vi "ServoControl_myrio_v3.vi"() -> ()   [LabVIEW 2019]
uses:
  <vilib>/Platform/TimedLoop/XDataNode/timing_clust.ctl
  <vilib>/Platform/TimedLoop/XDataNode/nitl_modes.ctl
  <vilib>/Platform/TimedLoop/XDataNode/wakeup.ctl
  <vilib>/Instr/_visa.llb/VISA Configure Serial Port (Instr).vi
  <vilib>/platform/TimedLoop/XDataNode/XDataNode.xnode
  <vilib>/Platform/TimedLoop/XDataNode/XDNodeRunTimeDep.lvlib
panel:
  in  "plot freq.":i32=100
  out "Position Graph":cluster{dbl[], dbl[]}[](graph)
  in  "stop":bool
  in  "const(f)/sine(t)":bool
  out "iteration":i32
  out "time":dbl
  out "sine position":dbl
  in  "Period":i64=5
  out "Position Chart":cluster{dbl, dbl}(graph)
  out "read from visa":string
  out "write to visa":string
  in  "VISA resource name":refnum<visa-resource-name>
  in  "baud rate (9600)":u32=500000
  in  "stop":bool
  out "read buffer 2":string
  in  "write buffer":string
  in  "Boolean 2":bool
  in  "const posotion":dbl
  out "error out":errorcluster
  # "white:write\nred:read"
  # "visa setting"
  # "measure time"
  # "status setting"
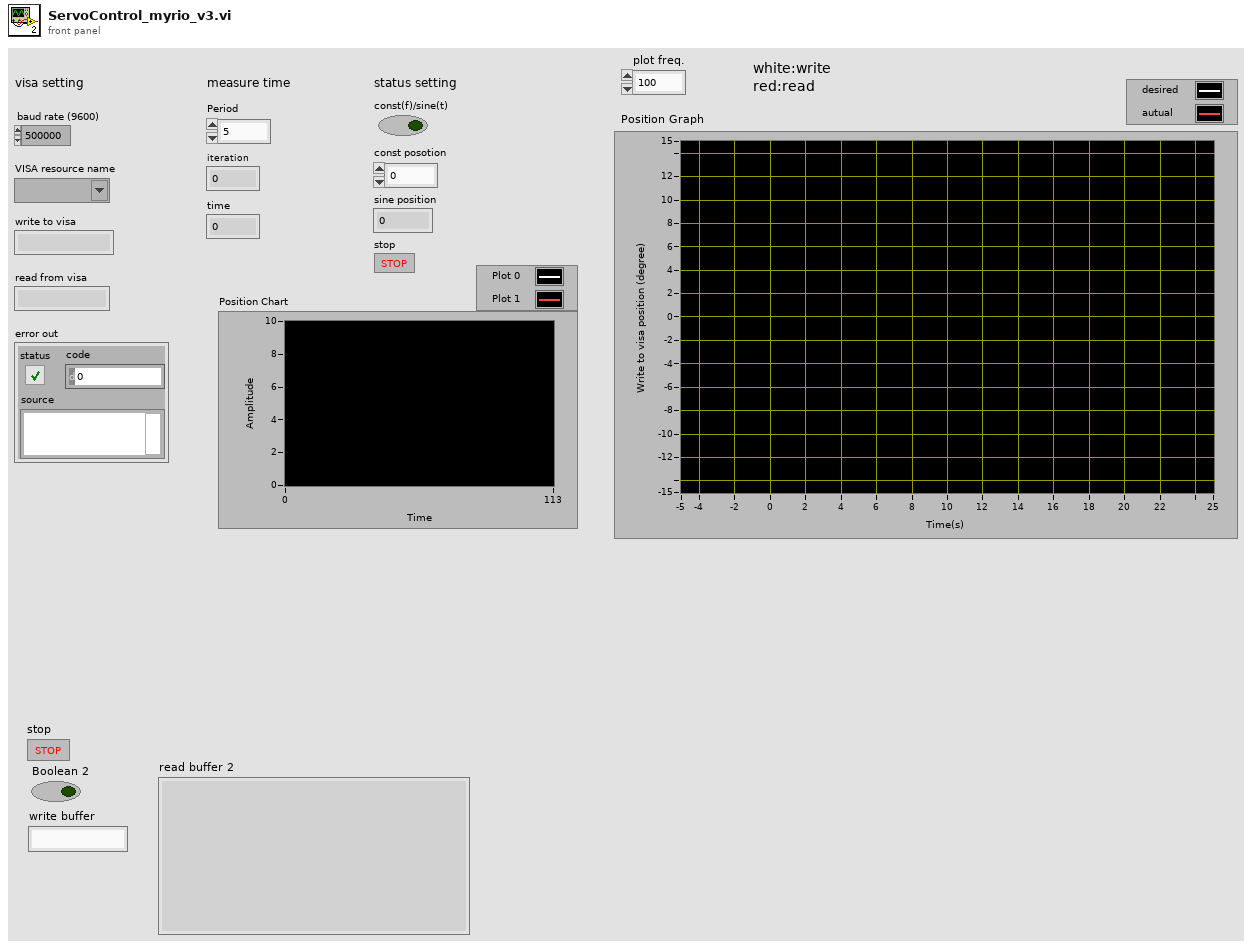
[diagram p1: front panel]
types:
  T1 = typedef "XDNodeRunTimeDep.lvlib/timing_clust.ctl" = cluster{"Expected End [f-1]":u64, "Actual End [f-1]":u64, "Finished Late? [f-1]":bool, "Expected End [i-1]":u64, "Actual End [i-1]":u64, "Finished Late? [i-1]":bool, "Expected Start [i]":u64, "Actual Start [i]":u64, "Expected Start [f]":u64, "Actual Start [f]":u64, "Source Name":string, "Structure Name":string, "Period":i64, "Deadline":i64, "Offset":i64, "Start":i64, "Priority":i32, "Timeout":i32, "Mode":T2, "Wakeup Reason":T3, "Error":errorcluster, "Source Type":string, "Secondary Source Type":string, "Global End Time":u64, "Global Start Time":u64, "Frame Duration":u64, "Iteration Duration":u64, "Assigned CPU":i32, "I/O Scan Engine Mode":u32}
  T2 = typedef "XDNodeRunTimeDep.lvlib/nitl_modes.ctl" = enum32{"No Change", "Process missed periods, maintain original phase", "Discard missed periods, maintain original phase", "Process missed periods, ignore original phase", "Discard missed periods, ignore original phase"}
  T3 = typedef "XDNodeRunTimeDep.lvlib/wakeup.ctl" = enum32{"Normal", "Aborted", "Asynchronous wakeup", "Timing source error", "Timed loop error", "Timeout"}
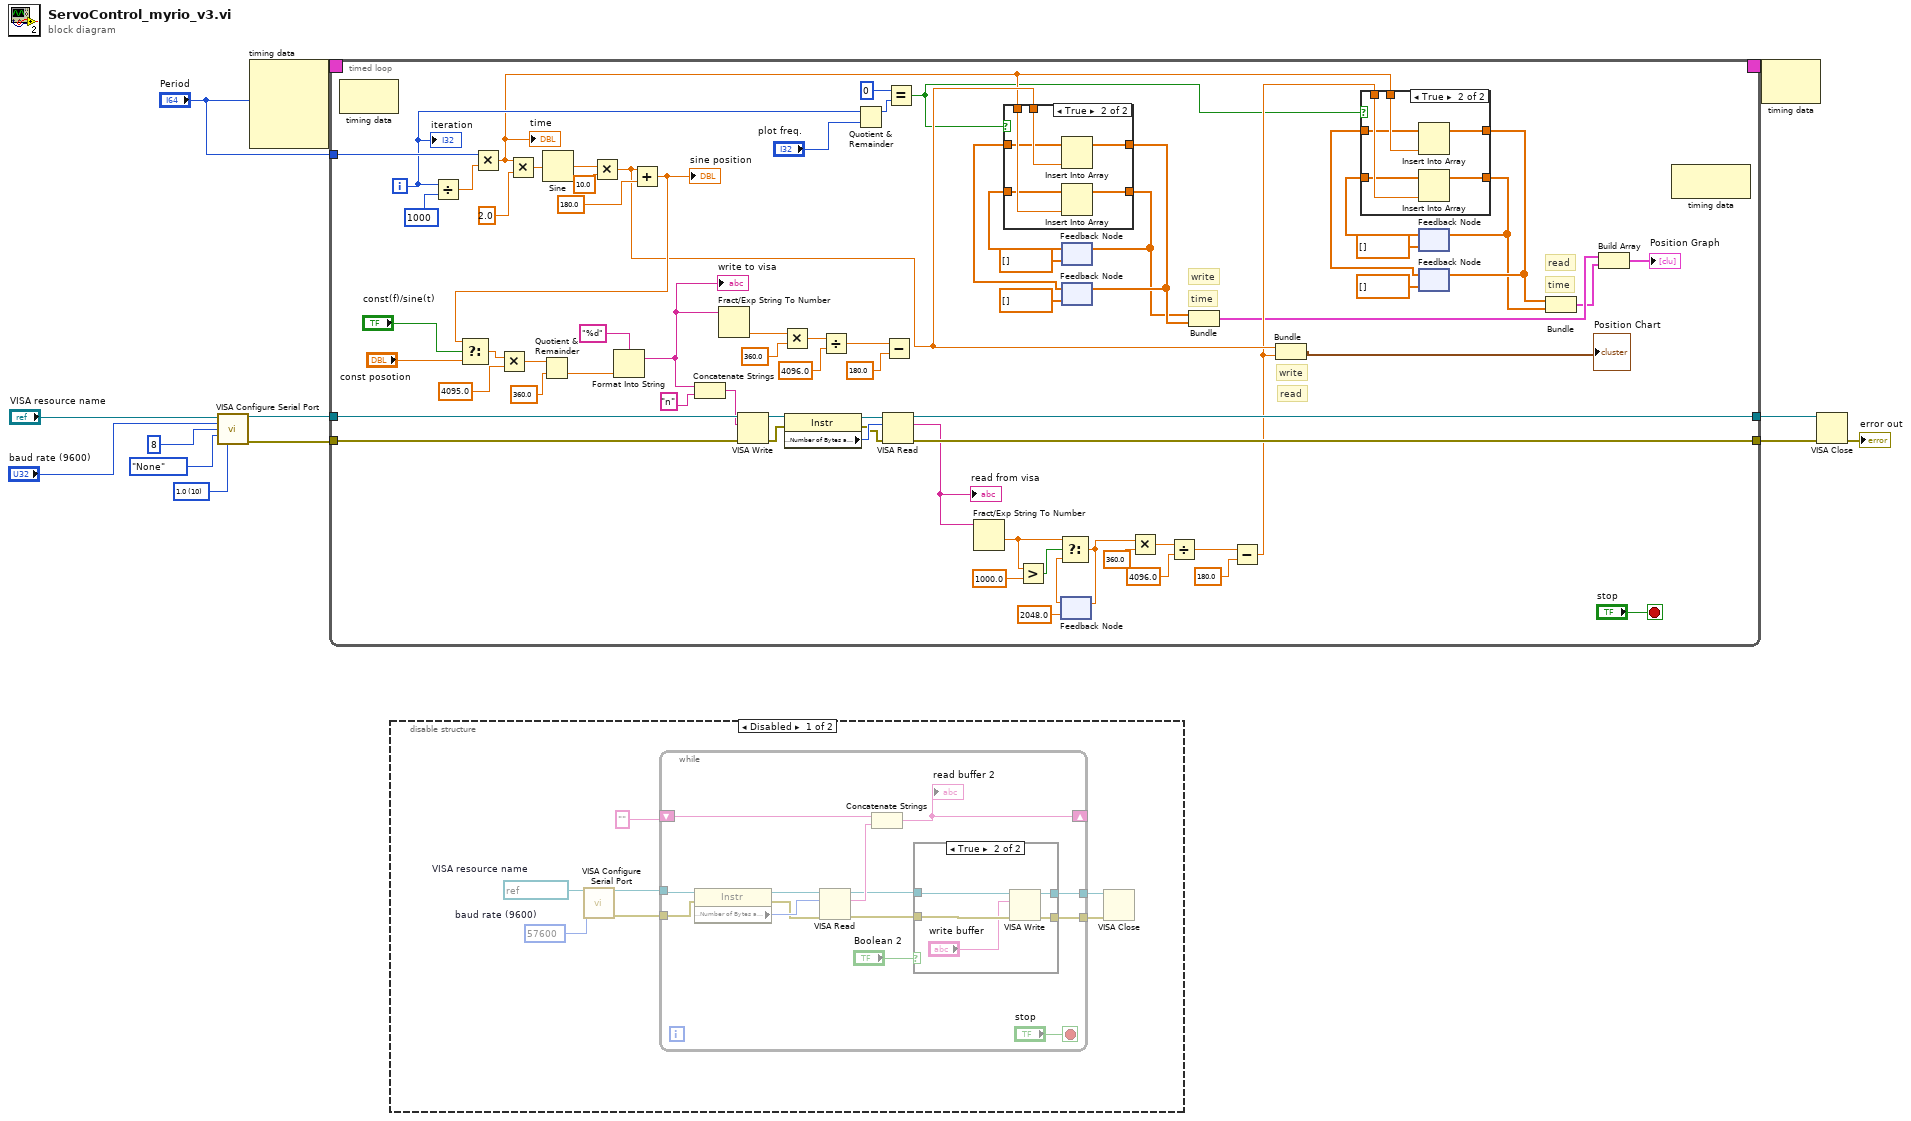
[diagram p0: block diagram]
diagram:
  w10 = u16 10 items=["1.0"=10, "1.5"=15, "2.0"=20] ("stop bits (10: 1 bit)")
  n1 = call-poly "VISA Configure Serial Port"("VISA resource name"="VISA resource name", "baud rate (9600)"="baud rate (9600)", "data bits (8)"=u16 8, "parity (0:none)"=enum16{"None", "Odd", "Even", "Mark", "Space"}."None", "stop bits (10: 1 bit)"=w10) -> ("VISA resource name out"=w9:refnum<visa-resource-name>, "error out"=w8:errorcluster)  [unwired: 9 in]
  n2 = node-c288("Period") -> (w3:T1)  [unwired: 3 in]
  n3 = timed-loop {
    timing: w3 -> [_]
    timing-out: [_] -> w2
    tunnel: "Period" -> [w55]
    tunnel: w8 -> [w84]
    tunnel: [w82] -> w6
    tunnel: w9 -> [w85]
    tunnel: [w83] -> w7
    i -> [w42]
    stop <- "stop" stop-if-true
    # "time"
    # "read"
    # "time"
    # "write"
    # "read"
    # "write"
    n4 = node-c288() -> ()  [unwired: 1 in, 1 out]
    n5 = Divide(x=w42, y=i64 1000) -> (x/y=w57:dbl)
    n6 = Multiply(x=w55, y=w57) -> (x*y=w22:dbl)
    "time" <- w22
    n7 = Multiply(x=w22, y=2.0) -> (x*y=w60:dbl)
    n8 = Sine(x=w60) -> (sin(x)=w39:dbl)
    n9 = Multiply(x=w39, y=10.0) -> (x*y=w27:dbl)
    n10 = Add(x=w27, y=180.0) -> (x+y=w53:dbl)
    "sine position" <- w53
    n11 = Select(t=w53, s="const(f)/sine(t)", f="const posotion") -> (s? t:f=w51:dbl)
    n12 = Multiply(x=w51, y=4095.0) -> (x*y=w79:dbl)
    n13 = Quotient & Remainder(x=w79, y=360.0) -> (floor(x/y)=w77:dbl)  [unwired: 1 out]
    n14 = Format Into String(format string="%d", w77) -> (resulting string=w69:string)  [unwired: 2 in, 1 out]
    "write to visa" <- w69
    n15 = Concatenate Strings(w69, "n" ("string")) -> (w81:string)
    n16 = Fract/Exp String To Number(string=w69) -> (number=w68:dbl)  [unwired: 3 in, 1 out]
    n17 = VISA Write(VISA resource name=w85, write buffer=w81, error in (no error)=w84) -> (VISA resource name out=w37:refnum<visa-resource-name>, error out=w36:errorcluster)  [unwired: 1 out]
    n18 = Multiply(x=w68, y=360.0 ("x")) -> (x*y=w66:dbl)
    n19 = property class="Instr"(reference=w37, error in=w36) -> (reference out=w34:refnum<visa-resource-name>, error out=w33:errorcluster, "Serial Settings:Number of Bytes at Serial Port"=w35:u32)
    n20 = Divide(x=w66, y=4096.0) -> (x/y=w72:dbl)
    n21 = Quotient & Remainder(x=w42, y="plot freq.") -> (x-y*floor(x/y)=w45:i32)  [unwired: 1 out]
    n22 = VISA Read(VISA resource name=w34, byte count=w35, error in (no error)=w33) -> (VISA resource name out=w83:refnum<visa-resource-name>, read buffer=w70:string, error out=w82:errorcluster)  [unwired: 1 out]
    "read from visa" <- w70
    n23 = Subtract(x=w72, y=180.0) -> ()  [unwired: 1 out]
    n24 = Equal?(x=0, y=w45) -> (x = y?=w17:bool)
    n25 = Fract/Exp String To Number(string=w70) -> (number=w31:dbl)  [unwired: 3 in, 1 out]
    n26 = Greater?(x=w31, y=1000.0) -> (0:w30:bool)
    n27 = feedback #1(2048.0) -> (w28:dbl)
    n28 = Select(t=w31, s=w30, f=w28) -> (s? t:f=w29:dbl)
    n29 = feedback-in #1(w29) -> ()
    n30 = feedback #2(dbl[] []) -> (w49:dbl[])
    n31 = feedback #3(dbl[] []) -> (w46:dbl[])
    n32 = case shown="True" w17 {
      tunnel: w27 -> [_ w101]
      tunnel: w22 -> [_ w100]
      tunnel: [w95 w99] -> w40
      tunnel: w49 -> [w95 w98]
      tunnel: [w94 w97] -> w41
      tunnel: w46 -> [w94 w96]
      frame False {
      }
      frame True {
        n33 = Insert Into Array(array=w96, new element=w101) -> (w97:dbl[])  [unwired: 1 in]
        n34 = Insert Into Array(array=w98, new element=w100) -> (w99:dbl[])  [unwired: 1 in]
      }
    }
    n35 = feedback-in #2(w40) -> ()
    n36 = feedback-in #3(w41) -> ()
    n37 = Multiply(x=w29, y=360.0 ("x")) -> (x*y=w61:dbl)
    n38 = Divide(x=w61, y=4096.0) -> (x/y=w63:dbl)
    n39 = Bundle(w40, w41) -> (w20:cluster{dbl[], dbl[]})  [unwired: 1 in]
    n40 = Subtract(x=w63, y=180.0) -> (x-y=w21:dbl)
    n41 = Bundle(w27, w21) -> (→"Position Chart":cluster{dbl, dbl})  [unwired: 1 in]
    n42 = feedback #4(dbl[] []) -> (w26:dbl[])
    n43 = feedback #5(dbl[] []) -> (w23:dbl[])
    n44 = case shown="True" w17 {
      tunnel: w22 -> [_ w93]
      tunnel: w21 -> [_ w92]
      tunnel: [w87 w91] -> w15
      tunnel: w26 -> [w87 w90]
      tunnel: [w86 w89] -> w16
      tunnel: w23 -> [w86 w88]
      frame False {
      }
      frame True {
        n45 = Insert Into Array(array=w88, new element=w93) -> (w89:dbl[])  [unwired: 1 in]
        n46 = Insert Into Array(array=w90, new element=w92) -> (w91:dbl[])  [unwired: 1 in]
      }
    }
    n47 = feedback-in #4(w15) -> ()
    n48 = feedback-in #5(w16) -> ()
    n49 = Bundle(w16, w15) -> (w19:cluster{dbl[], dbl[]})  [unwired: 1 in]
    n50 = Build Array(w20, w19) -> (→"Position Graph":cluster{dbl[], dbl[]}[])
    n51 = node-c288() -> ()  [unwired: 1 in, 1 out]
    "iteration" <- w42
  }
  n52 = disable-structure shown="Disabled" {
    frame Disabled {
      w109 = u32 57600  # baud rate (9600)
      w110 = refnum<visa-resource-name> "COM3"  # VISA resource name
      n53 = call-poly "VISA Configure Serial Port"("VISA resource name"=w110, "baud rate (9600)"=w109) -> ("VISA resource name out"=w108:refnum<visa-resource-name>, "error out"=w107:errorcluster)  [unwired: 12 in]
      n54 = while {
        tunnel: w108 -> [w123]
        tunnel: w107 -> [w122]
        shift-right: [w116] -> _
        shift-left: "" -> [w118]
        tunnel: [w113] -> w104
        tunnel: [w112] -> w105
        stop <- "stop" stop-if-true
        n55 = property class="Instr"(reference=w123, error in=w122) -> (reference out=w121:refnum<visa-resource-name>, error out=w119:errorcluster, "Serial Settings:Number of Bytes at Serial Port"=w120:u32)
        n56 = VISA Read(VISA resource name=w121, byte count=w120, error in (no error)=w119) -> (VISA resource name out=w115:refnum<visa-resource-name>, read buffer=w117:string, error out=w114:errorcluster)  [unwired: 1 out]
        n57 = Concatenate Strings(w118, w117) -> (w116:string)
        "read buffer 2" <- w116
        n58 = case shown="True" "Boolean 2" {
          tunnel: w115 -> [w126 w131]
          tunnel: w114 -> [w125 w130]
          tunnel: [w126 w129] -> w113
          tunnel: [w125 w128] -> w112
          frame False {
          }
          frame True {
            n59 = VISA Write(VISA resource name=w131, write buffer="write buffer", error in (no error)=w130) -> (VISA resource name out=w129:refnum<visa-resource-name>, error out=w128:errorcluster)  [unwired: 1 out]
          }
        }
      }
      n60 = VISA Close(VISA resource name=w104, error in (no error)=w105) -> ()  [unwired: 1 out]
    }
    frame Enabled {
    }
  }
  n61 = node-c288(w2) -> ()  [unwired: 1 out]
  n62 = VISA Close(VISA resource name=w7, error in (no error)=w6) -> (error out=→"error out":errorcluster)
